vi "Read Dispatcher Command.vi"(8 "error in (no error)":errorcluster, 9 "timeout in ms (0)":i32 format="%d ms", 11 "Dispatcher Interface in":refnum<class "Dispatcher Interface.lvclass">) -> (0 "error out":errorcluster, 2 "command":T1={"Command"=enum."Rx", "Parameters"={"arg1"=0, "arg2"=0}}, 3 "Dispatcher Interface out":refnum<class "Dispatcher Interface.lvclass">, 4 "# elements":u32)   [LabVIEW 2019, in "DSF Core.lvlib" / "Dispatcher Interface.lvclass"]
uses:
  Dispatcher Interface.lvclass
  C:/Dev/GitHub/niveristand-data-sharing-framework-custom-device/Core/Classes/Interface/Interface.lvclass
  Command Data.ctl
  Command.ctl
  Parameters.ctl
  Command Timeout.vi
  Interface.lvclass
  DSF Core.lvlib
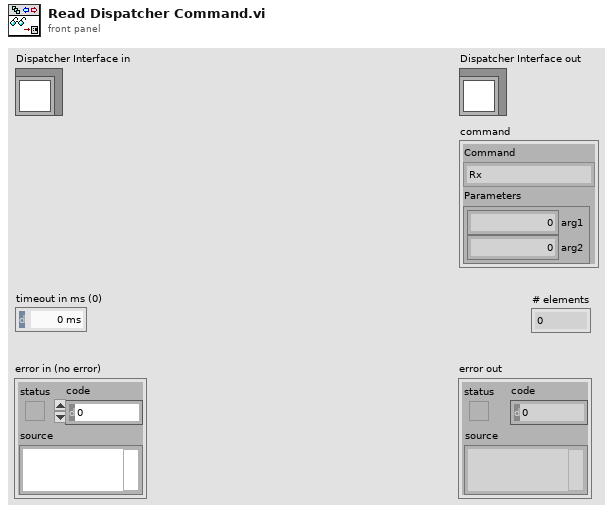
[diagram p1: front panel]
types:
  T1 = typedef "DSF Core.lvlib/Dispatcher Interface.lvclass/Command Data.ctl" = cluster{"Command":T2, "Parameters":T3}
  T2 = typedef "DSF Core.lvlib/Dispatcher Interface.lvclass/Command.ctl" = enum8{"Idle", "Start", "Rx", "Tx", "Set Inline Buffer", "Shutdown", "Error"}
  T3 = typedef "DSF Core.lvlib/Dispatcher Interface.lvclass/Parameters.ctl" = cluster{"arg1":u64, "arg2":u64}
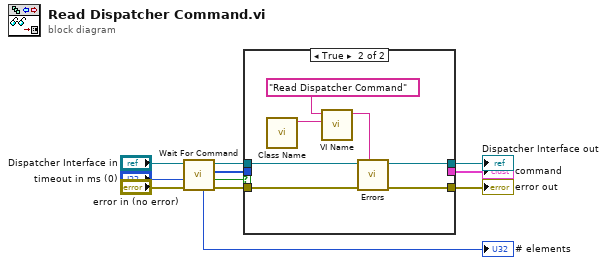
[diagram p0: block diagram]
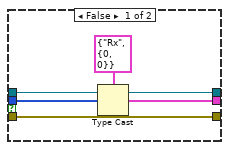
[diagram p2: hidden frame]
diagram:
  n1 = call "Wait For Command.vi"("error in (no error)"="error in (no error)", "timeout in ms (0)"="timeout in ms (0)", "Interface in"="Dispatcher Interface in") -> ("error out"=w2:errorcluster, "timed out?"=w5:bool, "command data"=w6:u8[], "Interface out"=w4:refnum<class "Dispatcher Interface.lvclass">, "# elements"=→"# elements":u32)  [unwired: 4 in]
  n2 = case shown="True" w5 {
    tunnel: [w14 _] -> w11
    tunnel: w6 -> [w13 _]
    tunnel: w4 -> [w16 w23]
    tunnel: [w16 w21] -> w3
    tunnel: w2 -> [w12 w22]
    tunnel: [w12 w20] -> w1
    frame False {
      n3 = Type Cast(type=T1 {"Command"=enum."Rx", "Parameters"={"arg1"=0, "arg2"=0}} ("Dispatcher Command"), x=w13) -> (*(type *) &x=w14:T1)
    }
    frame True {
      n4 = call "Class Name.vi"() -> ("class name"=w19:string)  [unwired: 11 in]
      n5 = call "VI Name.vi"("class name (\"\")"=w19, "vi name"="Read Dispatcher Command" ("error source vi name")) -> ("full VI name"=w17:string)  [unwired: 9 in]
      n6 = call-poly "Errors.vi"("error source vi name"=w17, "error in (no error)"=w22, "Interface in"=w23) -> ("error out"=w20:errorcluster, "Interface out"=w21:refnum<class "Dispatcher Interface.lvclass">)  [unwired: 7 in]
    }
  }
  "error out" <- w1
  "Dispatcher Interface out" <- w3
  "command" <- w11
